vi "Read DeviceDataModel[].vi"(8 "error in (no error)":errorcluster caption="错误输入（无错误）", 11 "Super Data Model输入":refnum<class "Super Data Model.lvclass">) -> (0 "error out":errorcluster caption="错误输出", 2 "DeviceDataModel[]":refnum<data-value>, 3 "Super Data Model输出":refnum<class "Super Data Model.lvclass">)   [LabVIEW 2013, in "Modbus Library - Advance.lvlib" / "Super Data Model.lvclass"]
uses:
  Super Data Model.lvclass
  Standard Data Model/Standard Data Model.lvclass
  Super Data Model.lvclass/Super Data Model.ctl
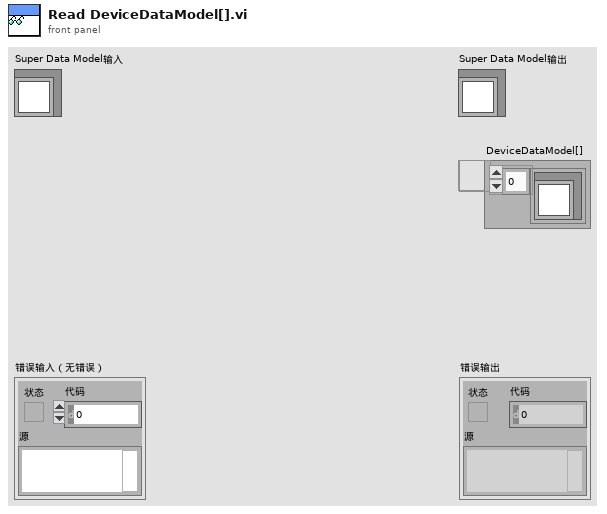
[diagram p1: front panel]
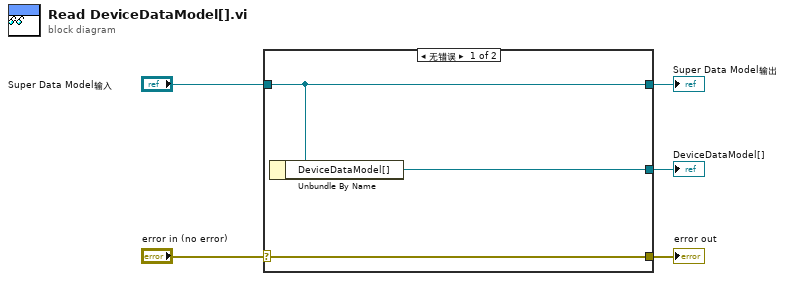
[diagram p0: block diagram]
diagram:
  n1 = case shown="无错误" "error in (no error)" {
    selector: "error in (no error)" -> [w8 w9]
    tunnel: [w8 w9] -> w4
    tunnel: [w7 w10] -> w2
    tunnel: "Super Data Model输入" -> [w7 w10]
    tunnel: [w6 _] -> w1
    frame No Error {
      n2 = Unbundle By Name(w7) -> ("DeviceDataModel[]"=w6:refnum<data-value>)
    }
    frame Error {
    }
  }
  "error out" <- w4
  "Super Data Model输出" <- w2
  "DeviceDataModel[]" <- w1
